vi "backwardPID.vi"(3 "NXT/EV3":T1) -> (1 "NXT/EV3 2":T1)   [LabVIEW 2016]
uses:
  <vilib>/NXT/Subs/LVHSConnector.ctl
  <vilib>/NXT/LegoClasses/BrickReference/BrickReference.lvclass
  <vilib>/NXT/Block Support/NXT_InputPort.ctl
  <vilib>/NXT/Block Support/NXT_OutputPort.ctl
  <vilib>/NXT/Dual Mode Library/Sensors/EV3_Gyro_Angle.vi
  <vilib>/NXT/NXTIO Xnodes/NXTIONodeSubVIs/NXTMoveMotors.vi
  <vilib>/NXT/NXTIO Xnodes/AddressXNode/NXTIOAddress.xnode
  <vilib>/NXT/NXTIO Xnodes/NXTIOXNode/NXTIO.xnode
panel:
  in  "Kp":sgl=2.0
  in  "Ki":sgl
  in  "Kd":sgl
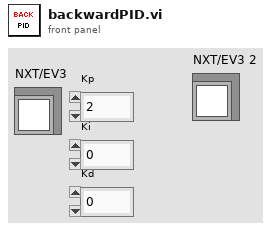
[diagram p1: front panel]
types:
  T1 = typedef "LVHSConnector.ctl" = refnum<class "BrickReference.lvclass">
  T2 = typedef "NXT_InputPort.ctl" = u32
  T3 = typedef "NXT_OutputPort.ctl" = u8
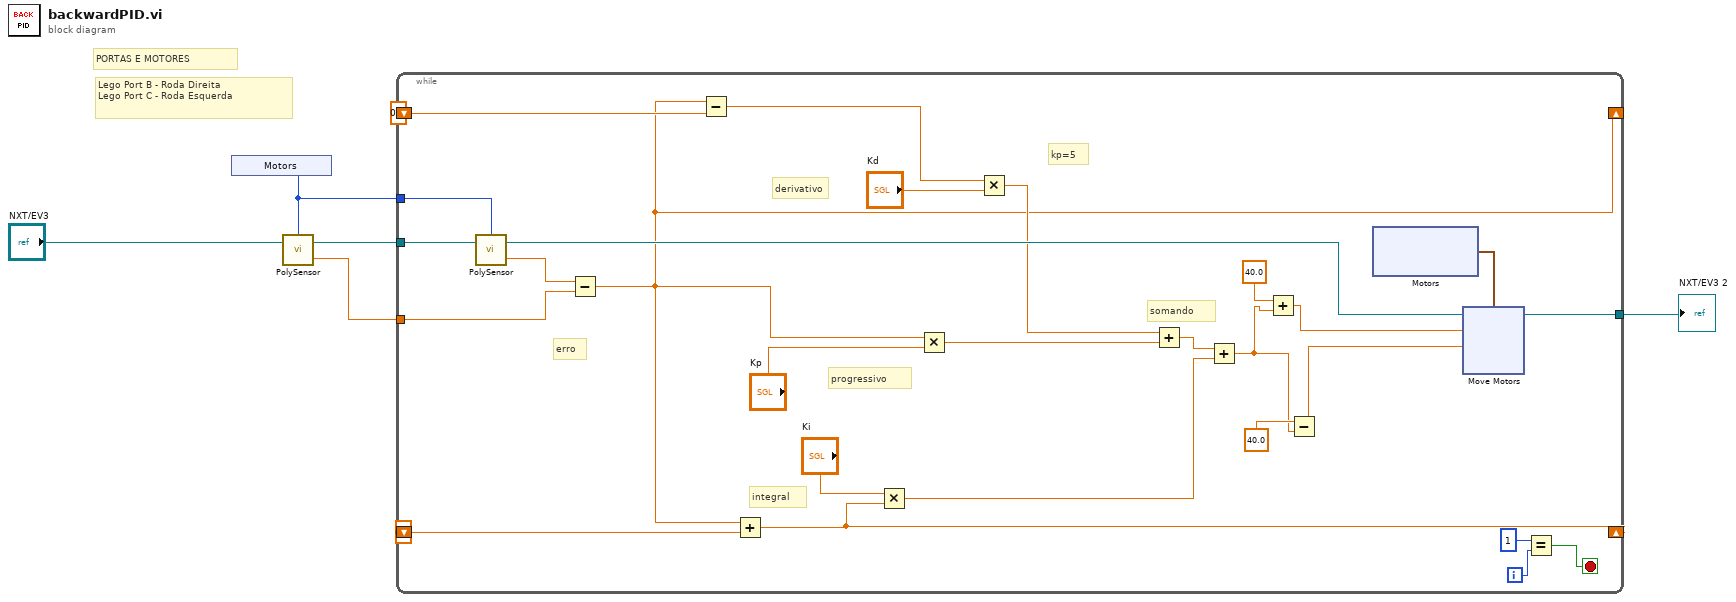
[diagram p0: block diagram]
diagram:
  # "Lego Port B - Roda Direita\nLego Port C - Roda Esquerda"
  # "PORTAS E MOTORES"
  n1 = xnode "Motors"() -> ("Sensor"=w3:T2)
  n2 = call-poly <vilib>:"PolySensor.vi"("NXT/EV3"="NXT/EV3", "Port (Port 1)"=w3) -> ("Degrees"=w2:sgl, "NXT/EV3"=w7:T1)  [unwired: 1 in]
  n3 = while {
    tunnel: w7 -> [w34]
    shift-right: [w26] -> _
    shift-left: sgl 0.0 -> [w28]
    shift-right: [w21] -> _
    shift-left: sgl 0.0 -> [w23]
    tunnel: w3 -> [w18]
    tunnel: w2 -> [w17]
    tunnel: [w11] -> w1
    i -> [w10]
    stop <- w8 stop-if-true
    # "kp=5"
    # "somando"
    # "erro"
    # "progressivo"
    # "integral"
    # "derivativo"
    n4 = call-poly <vilib>:"PolySensor.vi"("NXT/EV3"=w34, "Port (Port 1)"=w18) -> ("Degrees"=w22:sgl, "NXT/EV3"=w29:T1)  [unwired: 1 in]
    n5 = Subtract(x=w22, y=w17) -> (x-y=w21:sgl)
    n6 = Subtract(x=w21, y=w23) -> (x-y=w19:sgl)
    n7 = Add(x=w21, y=w28) -> (x+y=w26:sgl)
    n8 = Multiply(x="Ki", y=w26) -> (x*y=w25:sgl)
    n9 = Multiply(x=w21, y="Kp") -> (x*y=w31:sgl)
    n10 = Multiply(x=w19, y="Kd") -> (x*y=w24:sgl)
    n11 = Add(x=w24, y=w31) -> (x+y=w30:sgl)
    n12 = Add(x=w30, y=w25) -> (x+y=w12:sgl)
    n13 = Add(x=sgl 40.0, y=w12) -> (x+y=w15:sgl)
    n14 = Subtract(x=sgl 40.0, y=w12) -> (x-y=w14:sgl)
    n15 = xnode "Motors"() -> ("Motor"=w33:cluster{"Port":T3, "Port":T3})
    n16 = xnode "Move Motors"("Power/Speed 2"=w14, "Power/Speed 1"=w15, "Motors"=w33, "NXT/EV3"=w29) -> ("NXT/EV3"=w11:T1)
    n17 = Equal?(x=1, y=w10) -> (x = y?=w8:bool)
  }
  "NXT/EV3 2" <- w1
